vi "CSM - Send Message and Wait for Reply.vi"(6 "Response Timeout (-2 Using Global Settings)":i32=-2, 7 "Current Module (\"\" to Generate an ID)":string, 8 "Error In (No Error)":errorcluster, 9 "Target Module":string="Target", 10 "Arguments (\"\")":string, 11 "State":string="API State") -> (0 "error out":errorcluster, 2 "Response":string="DoA", 4 "Source CSM":string)   [LabVIEW 2017, in "Communicable State Machine.lvlib"]
doc: "Sends a synchronous message to the CSM and waits for a reply before continuing code execution.\n- If no reply message is received within the timeout, this VI returns a \"CSM Timeout Error\".\n- If the target module does not exist, this VI returns a \"Target Error\".\n\n\n> [!NOTE] <b>Synchronous Message</b>\n>\n> A synchronous message is a type of message. After a CSM sends a synchronous message, it pauses state transitions and waits for the callee to complete message processing. Synchronous messages are described via `-@`. A call from one JKISM module to another via a synchronous message is called a synchronous call.\n>\n> <b>Errors occurring at the Caller</b>:\n> - If the input target module is `\"\"`, a `NO Target Error` is generated.\n> - If the input module does not exist, a `Target Error` is generated.\n> - If the input module exists but does not complete processing within the specified time, a `Timeout Error` is generated.\n>\n> <b>Caller waits for return</b>:\n> - If the caller is a CSM module, it stays in the Parse State the Queue++ VI.\n> - If it is an API call, it stays in the calling VI, such as the CSM - Send Message and Wait for Reply VI.\n>\n> <b>Return</b>:\n> - <b>If the caller is a CSM module</b>:\n> - Normally, it enters the `Response` state to handle the return.\n> - If an error occurs at the caller, it causes the CSM state machine to enter the `Error Handler` module to handle the error.\n> - If an error occurs at the callee, this information is still the result of the message. It is handled in the `Response` state and can be obtained from Additional Information.\n> - <b>If it is an API call</b>:\n> - The Response output is the return.\n> - Errors occurring at both the caller and callee are merged into the error cluster output.\n\n\n> [!NOTE] <b>CSM Synchronous Message Global Timeout</b>\n>\n> - When performing CSM inter-module communication or using the VI that sends synchronous messages, the default timeout is -2, which uses the globally configured timeout.\n> - The global timeout can be set to other positive values using the CSM - Set TMO of Sync-Reply VI to override the global setting.\n> - The global timeout only applies to synchronous calls. Asynchronous calls are unaffected.\n\n\n> [!NOTE] <b>CSM Message Target Module Description</b>\n>\n> In Normal Mode, the target module for a CSM message is the specified module name.\n> System-level modules start with a `.` in their name. The target module for a CSM message includes the `.` in the name. For example, if the requested module name is `.System`, the target module for the CSM message is `.System`.\n> In Worker Mode, the target module for a CSM message can only be the overall module name, not the node name. For example, if the requested module name is `Worker#`, the target module for the CSM message is `Worker`.\n> In Chain of Responsibility Mode, the target module for a CSM message can only be the overall module name, not the node name. For example, if the requested module name is `Chain$1`, the target module for the CSM message is `Chain`.\n> In Chain of Responsibility Mode, a message is routed directly based on handling capability and priority (smaller number = higher priority) and is not passed sequentially across nodes.\n\n\n-- <b>Controls</b> --\n- <b>Current Module (\"\" to Generate an ID)</b>: Name of the current module. If empty, a temporary ID is generated for debugging purposes to identify the location.\n- <b>State</b>: Message string.\n- <b>Arguments (\"\")</b>: Message arguments.\n- <b>Target Module</b>: Target CSM module name.\n- <b>Response Timeout (-2 Using Global Settings)</b>: Timeout setting for waiting for a reply. The default is 5000 ms.\n\n-- <b>Indicators</b> --\n- <b>Response</b>: Returned response.\n- <b>Source CSM</b>: Name of the CSM module that sourced the returned response. In Worker Mode or Chain of Responsibility Mode, this output returns the name of the node."
uses:
  Communicable State Machine.lvlib
  CSM - Message Type.ctl
  _Support/GlobalEvent/LogFilter/LogFilter.lvclass/LogFilter.ctl
  _Support/CSMQ/_CSMObj-Message Check.vi
  _Support/CSMQ/_CSMObj-Enqueue Cross-Module Message.vi
  _Polymophic/Build Synchronous Message with Arguments.vi
  CSM - Make String Arguments Safe.vi
  _Support/CSMQ/_CSMOFGV Get.vi
  _Support/GlobalEvent/GEvt-Valid Subscribers.vi
  _Support/ChangeFlag/FlagInstance-GEvt Refs.vi
  _Support/GlobalEvent/GEvt-Convert Filter Rules - v1.2.vi
  _Support/ChangeFlag/FlagInstance-GEvt Filter.vi
  _Support/GlobalEvent/GEvt-Generate with Rule Check.vi
  _Shared/CSM - System States.vi
  _Support/Priority Queue/Enqueue Element.vi
  _Support/Message/Parse State with Arguments String.vi
  CSM - Keywords.vi
  _Support/ChangeFlag/ChangeFlag-Read.vi
  _Support/GlobalEvent/LogFilter/SettingVIs/Set Global CSM Filter.vi
  _Support/GlobalEvent/LogFilter/SettingVIs/Set Global LogType Filter.vi
  _Support/GlobalEvent/LogFilter/SettingVIs/Set Global State Filter.vi
  _Support/GlobalEvent/LogFilter/SettingVIs/Set CSM LogType Filter.vi
  _Support/GlobalEvent/LogFilter/SettingVIs/Set CSM State Filter.vi
  _Support/GlobalEvent/LogFilter/SettingVIs/Set Global StateType Filter.vi
  _Support/GlobalEvent/LogFilter/SettingVIs/Set CSM StateType Filter.vi
  _Support/GlobalEvent/LogFilter/SettingVIs/Set Periodic Log Filter.vi
  _Support/GlobalEvent/LogFilter/SettingVIs/Set CSM Broadcast Filter.vi
  _Support/GlobalEvent/LogFilter/SettingVIs/Set Global Broadcast Filter.vi
  _Support/GlobalEvent/LogFilter/SettingVIs/Set Global UserLog Filter.vi
  _Support/GlobalEvent/LogFilter/SettingVIs/Set CSM UserLog Filter.vi
  _Support/GlobalEvent/LogFilter/LogFilter - Check.vi
  _Support/GlobalEvent/LogFilter/CheckVIs/Group Check - LogType.vi
  _Support/GlobalEvent/LogFilter/CheckVIs/Group Check - CSM.vi
  _Support/GlobalEvent/LogFilter/CheckVIs/Group Check - State.vi
  _Support/GlobalEvent/LogFilter/CheckVIs/CSM Check - LogType.vi
  _Support/GlobalEvent/LogFilter/CheckVIs/CSM Check - State.vi
  _Support/GlobalEvent/LogFilter/CheckVIs/CSM Check - StateType.vi
  _Support/GlobalEvent/LogFilter/CheckVIs/Group Check - StateType.vi
  _Support/GlobalEvent/LogFilter/CheckVIs/CSM Check - Broadcast.vi
  _Support/GlobalEvent/LogFilter/CheckVIs/Group Check - Broadcast.vi
  _Support/GlobalEvent/LogFilter/CheckVIs/Group Check - UserLog.vi
  _Support/GlobalEvent/LogFilter/CheckVIs/CSM Check - UserLog.vi
  _Support/GlobalEvent/LogFilter/Support/Log State Type.vi
  _Support/CSMKVMap/CSMKVMap-Read.vi
  _Support/Error/CSM Not Allowed Message.vi
  _Support/CSMQ/_CSMOFGV(lvlibp).vi
  _Support/GlobalEvent/FGV-GEvt Filter Rules(lvlibp).vi
  _Support/ChangeFlag/ChangeFlagDB.vi
  _Support/GlobalEvent/FGV-GlobalEventQueues(lvlibp).vi
  _Support/GlobalEvent/FGV-GlobalEventRef(lvlibp).vi
  _Support/GlobalEvent/LogFilter/LogFilter.lvclass
  _Shared/CSM Shared.lvlib
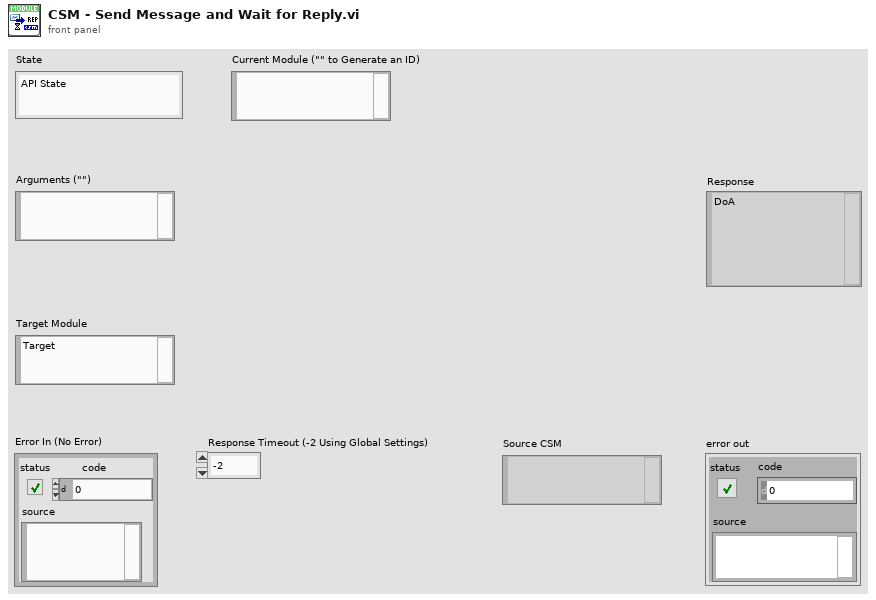
[diagram p1: front panel]
types:
  T1 = typedef "Communicable State Machine.lvlib/CSM - Message Type.ctl" = enum16{"Async", "Async without Reply", "Sync"}
  T2 = typedef "Communicable State Machine.lvlib/GEvt-Refs.ctl" = cluster{"Event":refnum<user-event>, "Queues":refnum<queue>[], "Valid":bool}
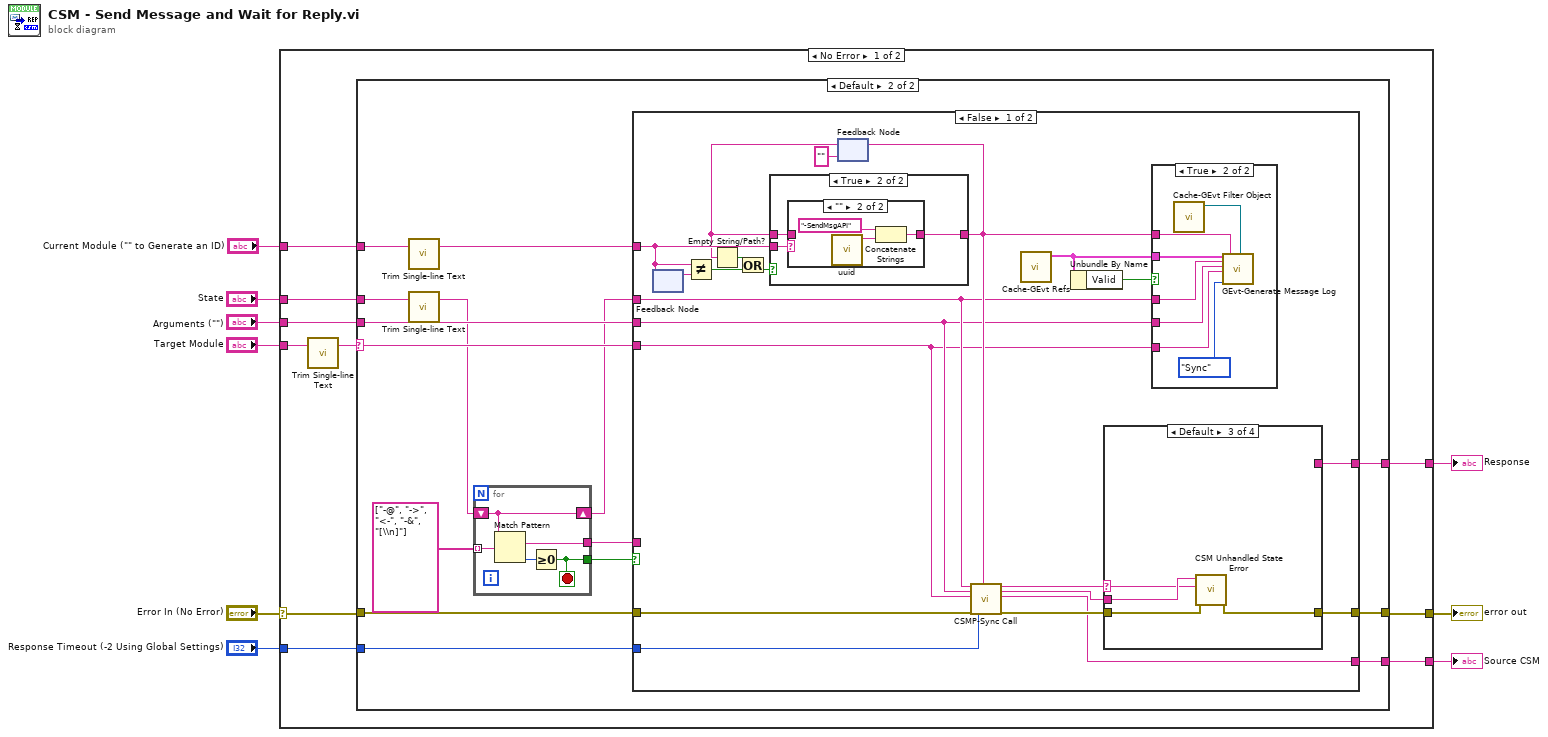
[diagram p0: block diagram]
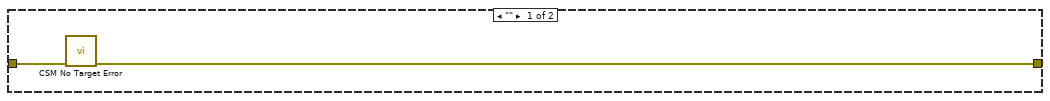
[diagram p2: hidden frame]
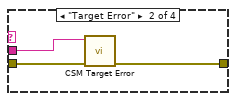
[diagram p7: hidden frame]
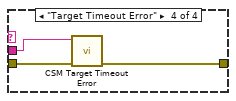
[diagram p8: hidden frame]
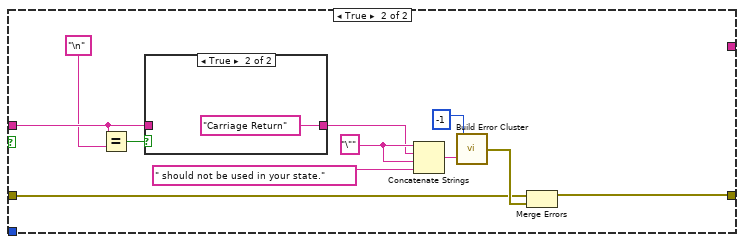
[diagram p9: hidden frame]
diagram:
  n1 = case shown="No Error" "Error In (No Error)" {
    selector: "Error In (No Error)" -> [w18 w103]
    tunnel: "State" -> [w19 _]
    tunnel: "Response Timeout (-2 Using Global Settings)" -> [w17 _]
    tunnel: [w13 w103] -> w6
    tunnel: [w16 _] -> w5
    tunnel: "Target Module" -> [w15 _]
    tunnel: "Arguments (\"\")" -> [w14 _]
    tunnel: "Current Module (\"\" to Generate an ID)" -> [w11 _]
    tunnel: [w10 _] -> w1
    frame No Error {
      n2 = call "Trim Single-line Text.vi"("single-line text"=w15) -> ("trimed text"=w12:string)  [unwired: 2 in]
      n3 = case shown="Default" w12 {
        selector: w12 -> [_ w33]
        tunnel: w18 -> [w21 w36]
        tunnel: w17 -> [_ w35]
        tunnel: [_ w34] -> w16
        tunnel: w14 -> [_ w32]
        tunnel: [w20 w31] -> w13
        tunnel: w19 -> [_ w30]
        tunnel: w11 -> [_ w23]
        tunnel: [_ w25] -> w10
        frame "" {
          n4 = call "CSM No Target Error.vi"("error in (no error)"=w21) -> ("error out"=w20:errorcluster)  [unwired: 10 in]
        }
        frame Default {
          n5 = call "Trim Single-line Text.vi"("single-line text"=w23) -> ("trimed text"=w22:string)  [unwired: 2 in]
          n6 = call "Trim Single-line Text.vi"("single-line text"=w30) -> ("trimed text"=w24:string)  [unwired: 2 in]
          n7 = for {
            shift-right: [w102] -> w29
            shift-left: w24 -> [w102]
            tunnel: string[] ["-@", "->", "<-", "-&", "[\\n]"] -> [w101] mode=indexing
            tunnel: [w99] -> w27
            tunnel: [w98] -> w28
            stop <- w98 stop-if-true
            n8 = Match Pattern(string=w102, regular expression=w101) -> (match substring=w99:string, offset past match=w100:i32)  [unwired: 1 in, 2 out]
            n9 = Greater Or Equal To 0?(x=w100) -> (x >= 0?=w98:bool)
          }
          n10 = case shown="False" w28 {
            tunnel: w36 -> [w57 w91]
            tunnel: w35 -> [w56 _]
            tunnel: [w51 _] -> w34
            tunnel: w33 -> [w38 _]
            tunnel: w32 -> [w39 _]
            tunnel: [w53 w92] -> w31
            tunnel: w29 -> [w40 _]
            tunnel: w27 -> [_ w87]
            tunnel: w22 -> [w48 _]
            tunnel: [w50 _] -> w25
            frame False {
              n11 = feedback-in #1(w48) -> ()
              n12 = feedback #1() -> (w49:string)  [unwired: 1 in]
              n13 = Not Equal?(x=w48, y=w49) -> (x != y?=w47:bool)
              n14 = feedback #2("") -> (w44:string)
              n15 = Empty String/Path?(string/path=w44) -> (empty?=w43:bool)
              n16 = Or(x=w43, y=w47) -> (x .or. y?=w45:bool)
              n17 = case shown="True" w45 {
                tunnel: w44 -> [w58 w61]
                tunnel: w48 -> [_ w60]
                tunnel: [w58 w59] -> w41
                frame False {
                }
                frame True {
                  n18 = case shown="\"\"" w60 {
                    selector: w60 -> [w62 _]
                    tunnel: [w62 w63] -> w59
                    tunnel: w61 -> [_ _]
                    frame Default {
                    }
                    frame "" {
                      n19 = call "uuid.vi"() -> ("UUID"=w64:string)  [unwired: 11 in]
                      n20 = Concatenate Strings("-SendMsgAPI" ("Name (\"\" to Use UUID)"), w64) -> (w63:string)
                    }
                  }
                }
              }
              n21 = feedback-in #2(w41) -> ()
              n22 = call "CSMP-Sync Call.vi"("State"=w40, "Args"=w39, "Source/target"=w38, "Error In"=w57, "Response Timeout (-2 Using Global Settings)"=w56, "Module Name"=w41) -> ("State Out"=w55:string, "Args Out"=w52:string, "Source/target Out"=w50:string, "Error"=w54:errorcluster)  [unwired: 8 in, 2 out]
              n23 = call "Cache-GEvt Refs.vi"() -> ("CSM Global Log Ref"=w42:T2)  [unwired: 10 in, 1 out]
              n24 = Unbundle By Name(w42) -> ("Valid"=w37:bool)
              n25 = case shown="Default" w55 {
                selector: w55 -> [_ _ w78 _]
                tunnel: w54 -> [w74 w76 w80 w83]
                tunnel: [w74 w75 w79 w82] -> w53
                tunnel: w52 -> [w73 w77 w81 w84]
                tunnel: [w73 _ _ _] -> w51
                frame "Response" {
                }
                frame "Target Error" {
                  n26 = call "CSM Target Error.vi"("error in (no error)"=w76, "Arguments (As CSM Name)"=w77) -> ("error out"=w75:errorcluster)  [unwired: 9 in]
                }
                frame Default {
                  n27 = call "CSM Unhandled State Error.vi"("error in (no error)"=w80, "Undefined State"=w78, "CSM Name"=w81) -> ("error out"=w79:errorcluster)  [unwired: 8 in]
                }
                frame "Target Timeout Error" {
                  n28 = call "CSM Target Timeout Error.vi"("error in (no error)"=w83, "Arguments (As CSM Name)"=w84) -> ("error out"=w82:errorcluster)  [unwired: 9 in]
                }
              }
              n29 = case shown="True" w37 {
                tunnel: w42 -> [_ w71]
                tunnel: w41 -> [_ w70]
                tunnel: w40 -> [_ w69]
                tunnel: w39 -> [_ w68]
                tunnel: w38 -> [_ w67]
                frame False {
                }
                frame True {
                  n30 = call "Cache-GEvt Filter Object.vi"() -> ("CSM:LogFilter.lvclass"=w72:refnum<class "LogFilter.lvclass">)  [unwired: 11 in]
                  n31 = call "GEvt-Generate Message Log.vi"("CSM Global Log Event"=w71, "Current State"=w69, "Arguments"=w68, "Source Module"=w67, "Type"=CSM_-_Message_Type."Sync", "Name (\"\" to Use UUID)"=w70, "CSM:LogFilter.lvclass"=w72) -> ()  [unwired: 11 in, 2 out]
                }
              }
            }
            frame True {
              w89 = "\"" ("string")
              n32 = Equal?(x=w87, y="\n" ("regular expression")) -> (x = y?=w85:bool)
              n33 = case shown="True" w85 {
                tunnel: [w96 "Carriage Return" ("State")] -> w88
                tunnel: w87 -> [w96 _]
                frame False {
                }
                frame True {
                }
              }
              n34 = Concatenate Strings(w89, w88, w89, " should not be used in your state." ("String to Prepend to source (\"\")")) -> (w90:string)
              n35 = call "Build Error Cluster.vi"("String to Prepend to Source (\"\")"=w90, "Code"=-1 ("code")) -> ("error out"=w93:errorcluster)
              n36 = Merge Errors(w91, w93) -> (w92:errorcluster)
            }
          }
        }
      }
    }
    frame Error {
    }
  }
  "error out" <- w6
  "Response" <- w5
  "Source CSM" <- w1
